vi "VC Initialize Hardware References.vi"(8 "error in (no error)":errorcluster, 10 "Message Data":variant, 11 "Hardware Resources in":T1) -> (0 "error out":errorcluster, 3 "Hardware Resources out":T1)   [LabVIEW 2020, in "Valve Control.lvlib"]
doc: "Initialize the hardware references."
uses:
  Valve Control.lvlib
  AM Configuration.ctl
  support/Message Queue/Message Cluster.ctl
  support/Message Queue/Message Queue.lvlib
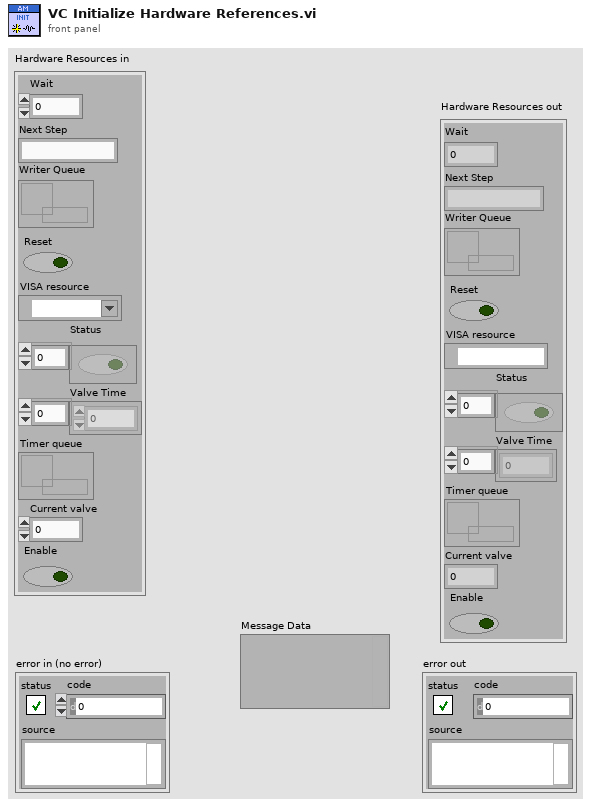
[diagram p1: front panel]
types:
  T1 = typedef "Valve Control.lvlib/AM Configuration.ctl" = cluster{"Wait":dbl, "Next Step":string, "Writer Queue":refnum<queue>, "Reset":bool, "VISA resource":refnum<visa-resource-name>, "Status":bool[], "Valve Time":dbl[], "Timer queue":refnum<queue>, "Current valve":i32, "Enable":bool}
  T2 = cluster{"Writer Queue":refnum<queue>, "Timeout":dbl[], "Status":bool[]}
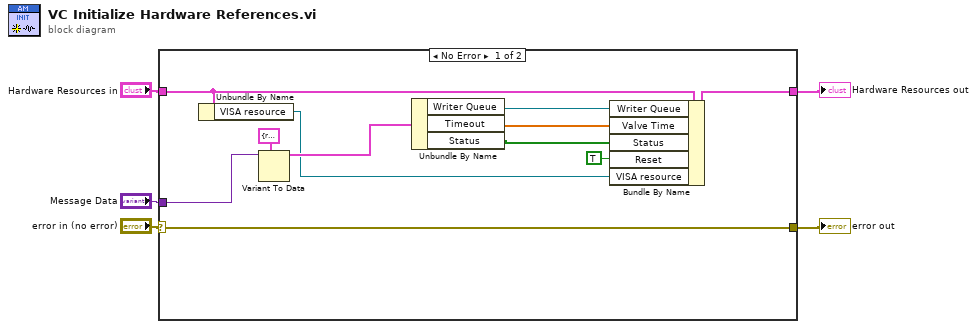
[diagram p0: block diagram]
diagram:
  n1 = case shown="No Error" "error in (no error)" {
    selector: "error in (no error)" -> [w7 w17]
    tunnel: [w7 w17] -> w4
    tunnel: "Hardware Resources in" -> [w9 w18]
    tunnel: [w15 w18] -> w1
    tunnel: "Message Data" -> [w16 _]
    frame No Error {
      n2 = Unbundle By Name(w9) -> ("VISA resource"=w8:refnum<visa-resource-name>)
      n3 = Variant To Data(type=T2 {"Writer Queue"=refnum, "Timeout"=[], "Status"=[]}, Variant=w16) -> (data=w14:T2)  [unwired: 1 in, 1 out]
      n4 = Unbundle By Name(w14) -> ("Writer Queue"=w13:refnum<queue>, "Timeout"=w12:dbl[], "Status"=w11:bool[])
      n5 = Bundle By Name(cluster=w9, "Writer Queue"=w13, "Valve Time"=w12, "Status"=w11, "Reset"=TRUE, "VISA resource"=w8) -> (w15:T1)
    }
    frame Error {
    }
  }
  "Hardware Resources out" <- w1
  "error out" <- w4
